vi "CleanUp.vi"(0 "object in":refnum<class "Application.lvclass">, 5 "error in (no error)":errorcluster) -> (14 "object out":refnum<class "Application.lvclass">, 19 "error out":errorcluster)   [LabVIEW 2023, in "Application.lvclass"]
uses:
  Application.lvclass
  Application.lvclass/Application.ctl
  AFG3022B_class/AFG3022B.lvclass
  AD2_SDK_class/AD2_SDK.lvclass
  CetoniPump_class/CetoniPump.lvclass
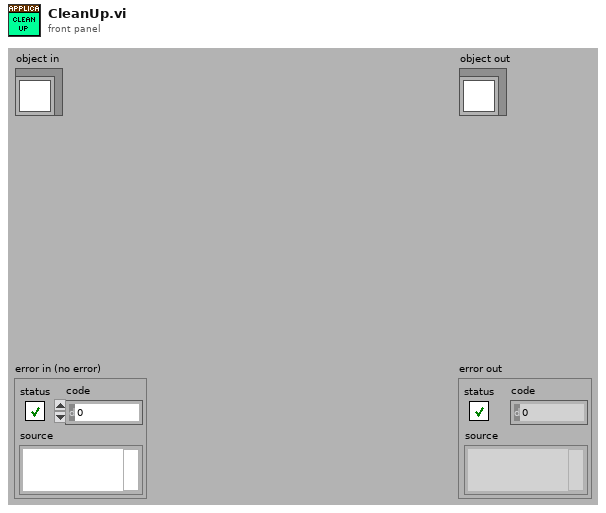
[diagram p1: front panel]
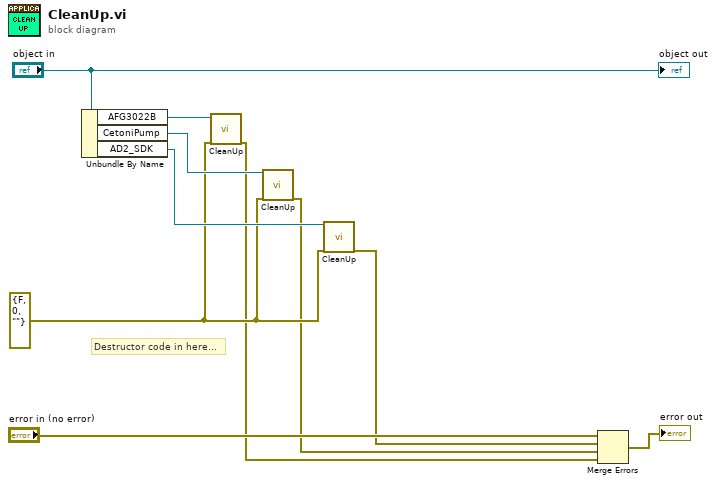
[diagram p0: block diagram]
diagram:
  w4 = errorcluster {"status"=FALSE, "code"=0, "source"=""} ("error in (no error)")
  # "Destructor code in here..."
  n1 = Unbundle By Name("object in") -> ("AFG3022B"=w7:refnum<class "AFG3022B.lvclass">, "CetoniPump"=w6:refnum<class "CetoniPump.lvclass">, "AD2_SDK"=w5:refnum<class "AD2_SDK.lvclass">)
  n2 = call-dynamic "CleanUp.vi"("object in"=w7, "error in (no error)"=w4) -> ("error out"=w3:errorcluster)  [unwired: 16 in, 1 out]
  n3 = call-dynamic "CleanUp.vi"("object in"=w6, "error in (no error)"=w4) -> ("error out"=w2:errorcluster)  [unwired: 16 in, 1 out]
  n4 = call-dynamic "CleanUp.vi"("object in"=w5, "error in (no error)"=w4) -> ("error out"=w1:errorcluster)  [unwired: 16 in, 1 out]
  n5 = Merge Errors("error in (no error)", w1, w2, w3) -> (→"error out":errorcluster)
  "object out" <- "object in"
